vi "Validate Hardware Custom Device API Version 1.vi"(8 "error in (no error)":errorcluster, 11 "Hardware Ref in":T1 format="%.0x") -> (0 "error out":errorcluster, 3 "Hardware Ref out":T1 format="%.0x")   [LabVIEW 2020, in "Routing and Faulting Hardware API.lvlib"]
uses:
  Routing and Faulting Hardware API.lvlib
  <vilib>/NI VeriStand/Custom Device API/Custom Device Item Ref.ctl
  <vilib>/NI VeriStand/Custom Device API/Custom Device API.lvlib
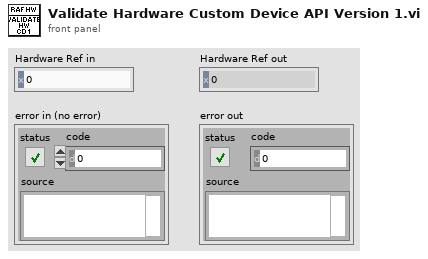
[diagram p1: front panel]
types:
  T1 = typedef "Custom Device API.lvlib/Custom Device Item Ref.ctl" = u64
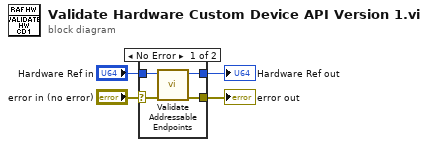
[diagram p0: block diagram]
diagram:
  n1 = case shown="No Error" "error in (no error)" {
    selector: "error in (no error)" -> [w7 w10]
    tunnel: [w6 w10] -> w2
    tunnel: [w5 w9] -> w3
    tunnel: "Hardware Ref in" -> [w8 w9]
    frame No Error {
      n2 = call "Validate Addressable Endpoints.vi"("error in (no error)"=w7, "Hardware Ref in"=w8) -> ("error out"=w6:errorcluster, "Hardware Ref out"=w5:T1)  [unwired: 8 in]
    }
    frame Error {
    }
  }
  "Hardware Ref out" <- w3
  "error out" <- w2
